vi "Position_Generic.vi"() -> ()   [LabVIEW 2013, in "GenericMotionCore.lvlib"]
uses:
  <instrlib>/GenericMotionCore/GenericMotionCore.lvlib
panel:
  in  "tickcount_pos":u32
  out "Moving(Generic)":bool
  in  "Position(Generic)":dbl[](array[numeric]) caption="Position" format="%.4f"
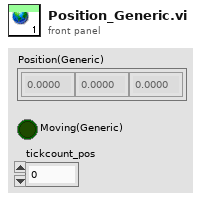
[diagram p1: front panel]
diagram:
